vi "processScanCommand.vi"(8 "error in (no error)":errorcluster, 10 "Queues":T5, 11 "FPGA VI Reference In":T4) -> (0 "error out":errorcluster, 1 "command queue status":T1, 3 "num calls":T3, 4 "num lines sent":u32, 5 "num new volumes":i32, 6 "current volume":T2, 7 "line volume nums":i32[](array[numeric]))   [LabVIEW 2010]
uses:
  internal_queues.ctl
  line_info.ctl
  volume_with_lines.ctl
  volume_info.ctl
  FPGA_ref.ctl
  <vilib>/rvi/interface/nirviMethod/nirviMethod.xnode
  <vilib>/rvi/interface/common/niFpgaNodeNameForErrorReporting.ctl
  <vilib>/rvi/errors/niLvFpgaWhatHappensToTopLevelVI.ctl
  FPGA scanInfo/scan message.ctl
  <vilib>/Utility/error.llb/Error Cluster From Error Code.vi
  <vilib>/rvi/errors/niLvFpgaAdjustHostInterfaceError.vi
  NiFpgaLv.dll
panel:
  # "140 kHz * 2 = 280/ms"
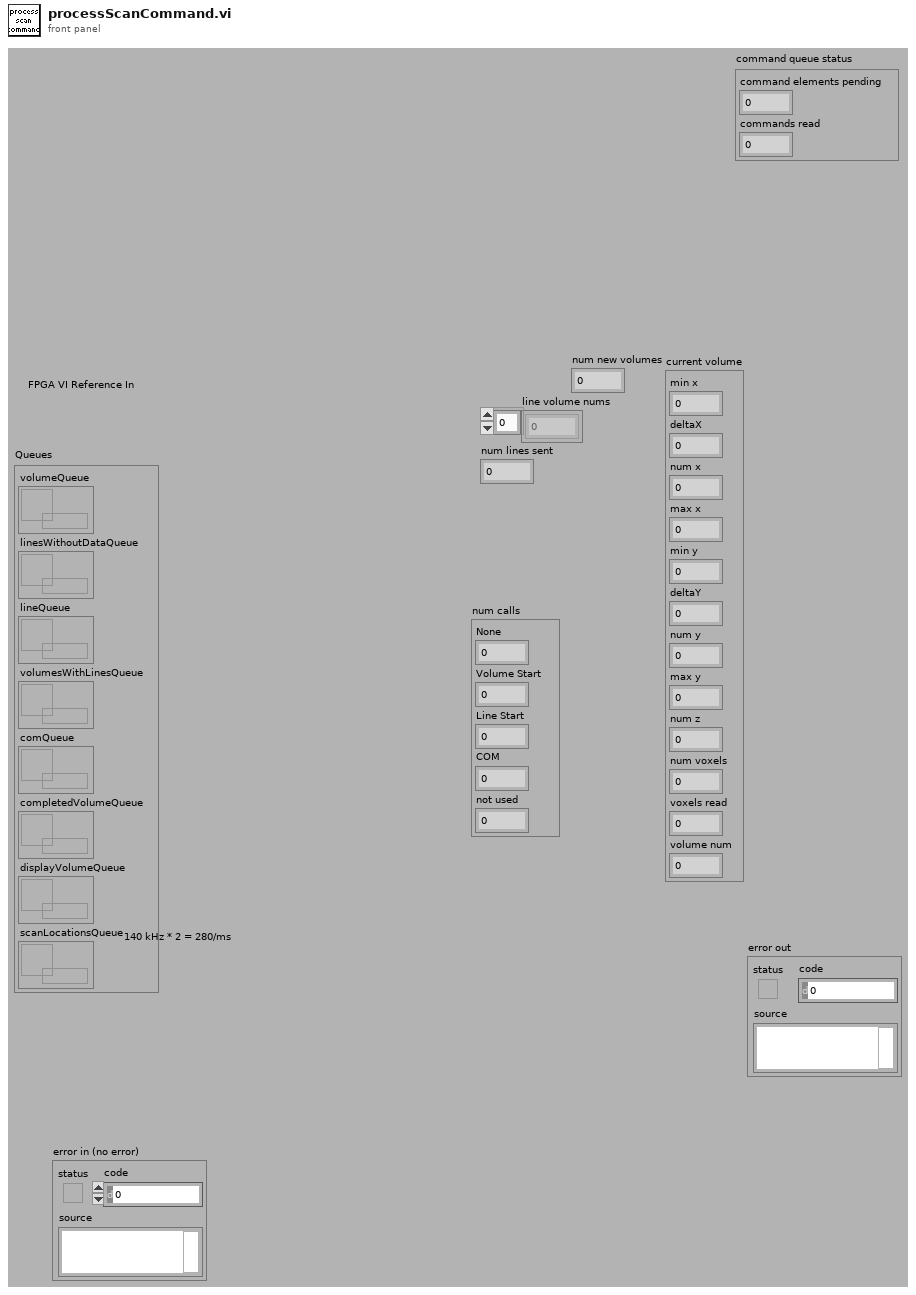
[diagram p1: front panel]
types:
  T1 = cluster{"command elements pending":u32, "commands read":u32}
  T2 = cluster{"min x":i16, "deltaX":dbl, "num x":u32, "max x":i16, "min y":i16, "deltaY":dbl, "num y":u32, "max y":i16, "num z":u32, "num voxels":u32, "voxels read":u32, "volume num":u32}
  T3 = cluster{"None":i32, "Volume Start":i32, "Line Start":i32, "COM":i32, "not used":i32}
  T4 = typedef "FPGA_ref.ctl" = refnum<k20>
  T5 = typedef "internal_queues.ctl" = cluster{"volumeQueue":refnum<queue>, "linesWithoutDataQueue":refnum<queue>, "lineQueue":refnum<queue>, "volumesWithLinesQueue":refnum<queue>, "comQueue":refnum<queue>, "completedVolumeQueue":refnum<queue>, "displayVolumeQueue":refnum<queue>, "scanLocationsQueue":refnum<queue>}
  T6 = cluster{"[0]":i32, "[1]":i32, "[2]":i32, "[3]":i32, "[4]":i32}
  T7 = typedef "scan message.ctl" = enum16{"NONE", "VOLUME START", "LINE START", "COM"}
  T8 = typedef "line_info.ctl" = cluster{"start X":i16, "start Y":i16, "start Z":i16, "end X":i16, "end Y":i16, "end Z":i16, "num z":u8, "voxel data":u32[], "volume num":u32, "line number":u16, "unused":u16}
  T9 = cluster{"Data[0]":i32, "Data[1]":i32, "Data[2]":i32, "Data[3]":i32, "Data[4]":i32}
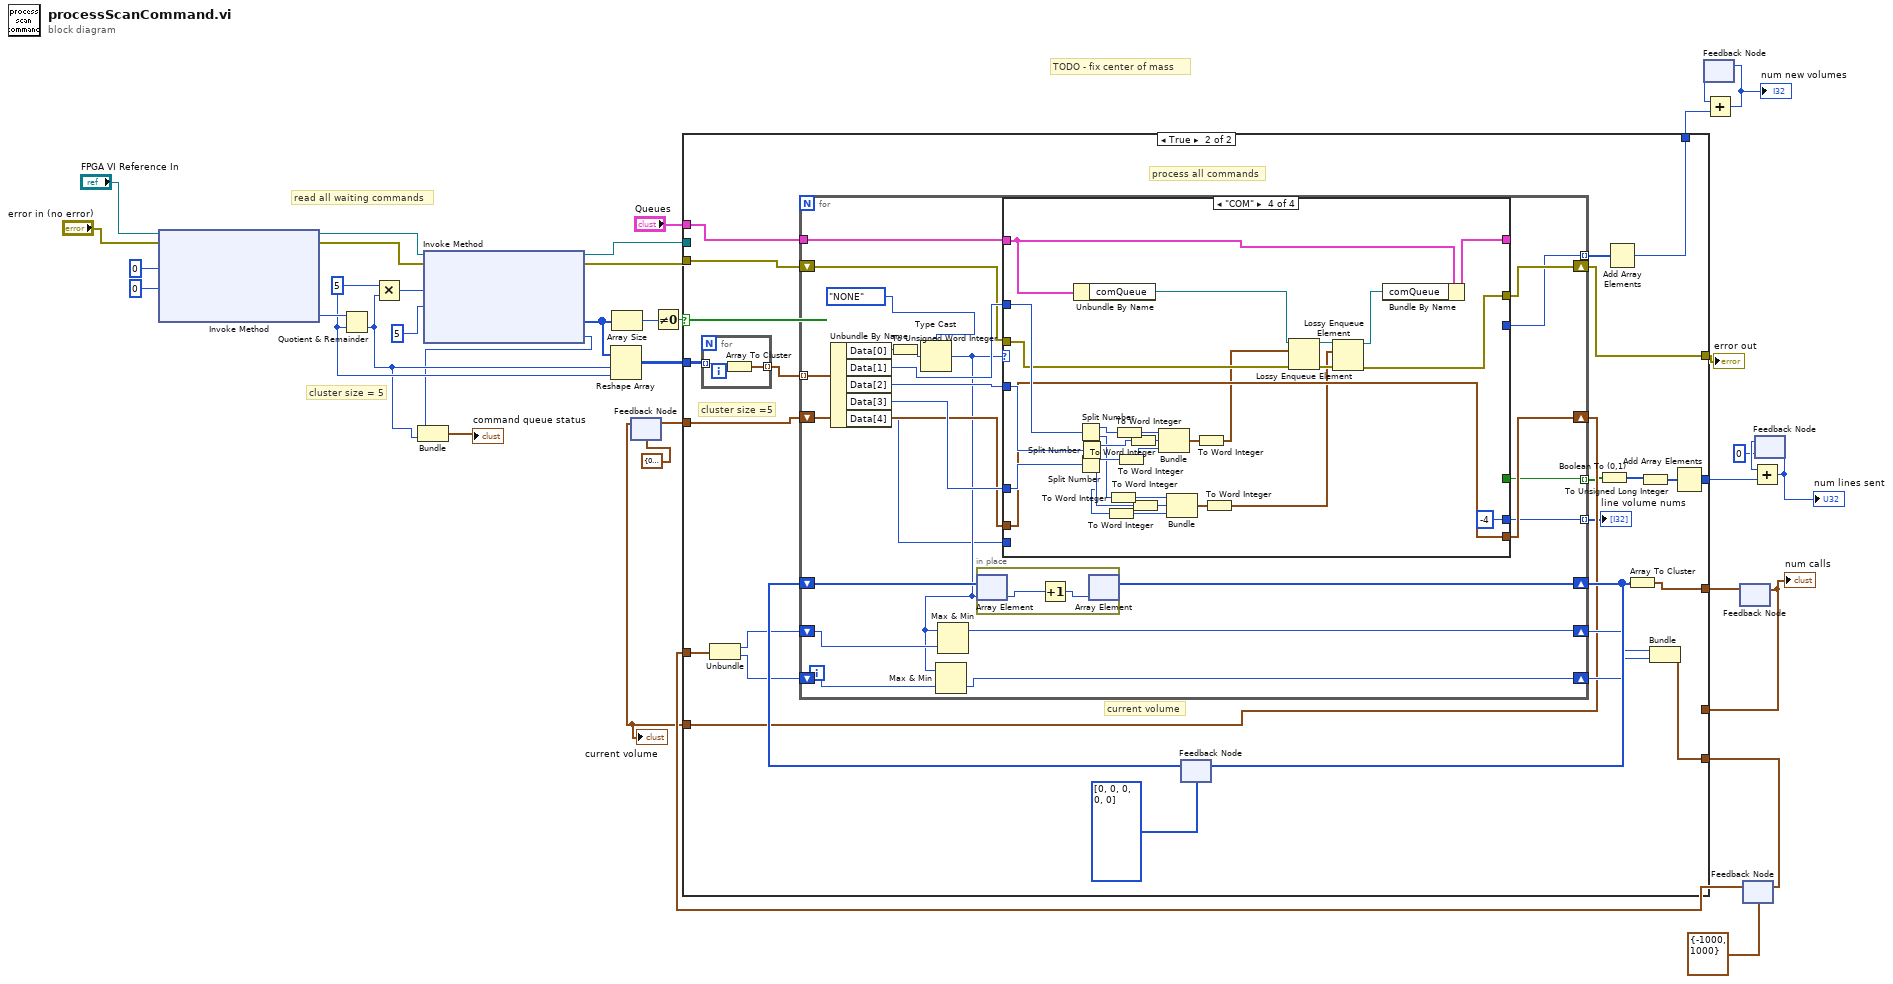
[diagram p0: block diagram]
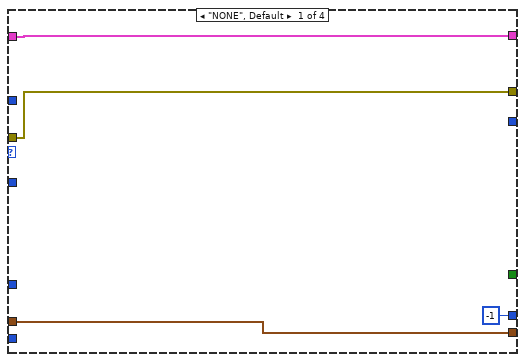
[diagram p3: hidden frame]
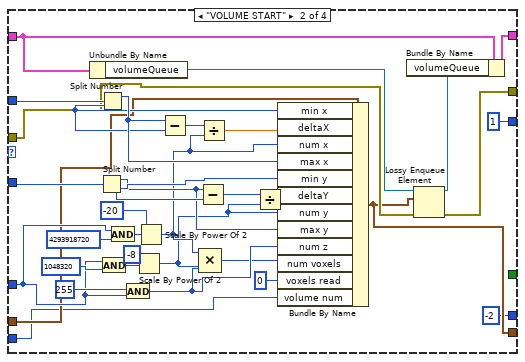
[diagram p4: hidden frame]
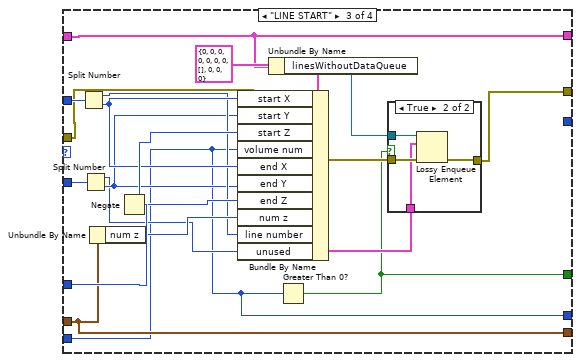
[diagram p5: hidden frame]
diagram:
  w24 = u32 5 ("Number of Elements")
  # "TODO - fix center of mass"
  # "read all waiting commands"
  # "cluster size = 5"
  n1 = xnode "Invoke Method"("FPGA VI Reference In"="FPGA VI Reference In", "error in"="error in (no error)", "Number of Elements"=u32 0, "Timeout (ms)"=0) -> ("FPGA VI Reference Out"=w22:T4, "error out"=w23:errorcluster, "Elements Remaining"=w25:u32)  [unwired: 1 out]
  n2 = Quotient & Remainder(x=w25, y=w24) -> (floor(x/y)=w6:u32)  [unwired: 1 out]
  n3 = Multiply(x=w24, y=w6) -> (x*y=w32:u32)
  n4 = xnode "Invoke Method"("FPGA VI Reference In"=w22, "error in"=w23, "Number of Elements"=w32, "Timeout (ms)"=5) -> ("FPGA VI Reference Out"=w33:T4, "error out"=w34:errorcluster, "Data"=w30:i32[], "Elements Remaining"=w5:u32)
  n5 = Bundle("Elements Remaining"=w5, w6) -> (→"command queue status":cluster{"Elements Remaining":u32, u32})  [unwired: 1 in]
  n6 = Reshape Array(w30, w6, w24) -> (w21:i32[][])
  n7 = Array Size(array=w30) -> (size(s)=w35:i32)
  n8 = feedback #1(T2 {"min x"=0, "deltaX"=0.0, "num x"=0, "max x"=0, "min y"=0, "deltaY"=0.0, "num y"=0, "max y"=0, "num z"=0, "num voxels"=0, "voxels read"=0, "volume num"=0} ("current volume")) -> (w9:T2)
  n9 = Not Equal To 0?(x=w35) -> (x != 0?=w31:bool)
  n10 = feedback #2() -> (w11:i32)  [unwired: 1 in]
  n11 = feedback #3() -> (w17:T6)  [unwired: 1 in]
  "num calls" <- w17
  n12 = feedback #4(cluster{i32, i32} {-1000, 1000}) -> (w16:cluster{i32, i32})
  n13 = case shown="True" w31 {
    tunnel: w34 -> [w40 w64]
    tunnel: w33 -> [_ _]
    tunnel: w21 -> [_ w63]
    tunnel: "Queues" -> [_ w61]
    tunnel: [w40 w46] -> w19
    tunnel: [w39 w57] -> w18
    tunnel: w17 -> [w39 _]
    tunnel: [w38 w54] -> w15
    tunnel: w16 -> [w38 w53]
    tunnel: [_ w49] -> w13
    tunnel: w9 -> [w37 w48]
    tunnel: [w37 w47] -> w8
    tunnel: [_ w41] -> w4
    frame False {
    }
    frame True {
      # "current volume"
      # "process all commands"
      # "cluster size =5"
      n14 = for {
        tunnel: w63 -> [w181] mode=indexing
        tunnel: [w180] -> w62 mode=indexing
        n15 = Array To Cluster(array=w181) -> (cluster=w180:T9)
      }
      n16 = Unbundle(w53) -> (w52:i32, w51:i32)
      n17 = feedback #5(i32[] [0, 0, 0, 0, 0]) -> (w60:i32[])
      n18 = for {
        tunnel: w62 -> [w67] mode=indexing
        shift-right: [w84] -> w46
        shift-left: w64 -> [w83]
        shift-right: [w81] -> w47
        shift-left: w48 -> [w80]
        shift-right: [w78] -> w58
        shift-left: w60 -> [w79]
        shift-right: [w76] -> w56
        shift-left: w52 -> [w75]
        shift-right: [w74] -> w55
        shift-left: w51 -> [w73]
        tunnel: [w72] -> w50 mode=indexing
        tunnel: w61 -> [w82]
        tunnel: [w66] -> w45 mode=indexing
        tunnel: [w65] -> w44 mode=indexing
        n19 = Unbundle By Name(w67) -> ("Data[0]"=w77:i32, "Data[1]"=w87:i32, "Data[2]"=w86:i32, "Data[3]"=w85:i32, "Data[4]"=w68:i32)
        n20 = To Unsigned Word Integer(number=w77) -> (unsigned 16bit integer=w70:u16)
        n21 = Type Cast(type=scan_message."NONE" ("Enum"), x=w70) -> (*(type *) &x=w71:T7)
        n22 = Max & Min(x=w71, y=w73) -> (min(x,y)=w74:i32)  [unwired: 1 out]
        n23 = Max & Min(x=w71, y=w75) -> (max(x,y)=w76:i32)  [unwired: 1 out]
        n24 = in-place {
          n25 = in-place-array #6(w79, w71) -> (w89:i32)
          n26 = Increment(x=w89) -> (x+1=w88:i32)
          n27 = in-place-array #6(w88) -> (w78:i32[])  [unwired: 1 out]
        }
        n28 = case shown="\"COM\"" w71 {
          tunnel: w87 -> [_ w127 w145 w178]
          tunnel: w86 -> [_ w126 w144 w177]
          tunnel: w85 -> [_ w122 w143 w176]
          tunnel: w82 -> [w93 w108 w138 w174]
          tunnel: w83 -> [w92 w110 w136 w171]
          tunnel: [w93 w106 w138 w173] -> _
          tunnel: [w92 w105 w135 w160] -> w84
          tunnel: [w91 w103 w141 w172] -> w81
          tunnel: w80 -> [w91 w104 w141 w172]
          tunnel: [_ 1 _ _] -> w72
          tunnel: w68 -> [_ w95 w129 _]
          tunnel: [-1 ("Data[4]") -2 ("Data[4]") w129 -4 ("Data[4]")] -> w66
          tunnel: [_ _ w128 _] -> w65
          frame "NONE", Default {
          }
          frame "VOLUME START" {
            n29 = Unbundle By Name(w108) -> ("volumeQueue"=w109:refnum<queue>)
            n30 = Split Number(x=w126) -> (hi(x)=w114:u16, lo(x)=w116:u16)
            n31 = Split Number(x=w127) -> (hi(x)=w119:u16, lo(x)=w118:u16)
            n32 = And(x=w122, y=u32 1048320) -> (x .and. y?=w98:u32)
            n33 = And(x=w122, y=u32 4293918720) -> (x .and. y?=w101:u32)
            n34 = And(x=u32 255, y=w122) -> (x .and. y?=w113:u32)
            n35 = Scale By Power Of 2(n=-8, x=w98) -> (x*2^n=w97:u32)
            n36 = Scale By Power Of 2(n=-20, x=w101) -> (x*2^n=w100:u32)
            n37 = Subtract(x=w119, y=w118) -> (x-y=w121:u16)
            n38 = Subtract(x=w114, y=w116) -> (x-y=w120:u16)
            n39 = Divide(x=w121, y=w100) -> (x/y=w117:dbl)
            n40 = Compound Arithmetic op=MULTIPLY(w100, w97, w113) -> (w112:u32)
            n41 = Divide(x=w120, y=w97) -> (x/y=w115:dbl)
            n42 = Bundle By Name(cluster=w104, "min x"=w118, "deltaX"=w117, "num x"=w100, "max x"=w119, "min y"=w116, "deltaY"=w115, "num y"=w97, "max y"=w114, "num z"=w113, "num voxels"=w112, "voxels read"=u32 0, "volume num"=w95) -> (w103:T2)
            n43 = Lossy Enqueue Element(queue=w109, element=w103, error in (no error)=w110) -> (queue out=w107:refnum<queue>, error out=w105:errorcluster)  [unwired: 2 out]
            n44 = Bundle By Name(cluster=w108, "volumeQueue"=w107) -> (w106:T5)
          }
          frame "LINE START" {
            n45 = Split Number(x=w145) -> (hi(x)=w132:u16, lo(x)=w133:u16)
            n46 = Split Number(x=w144) -> (hi(x)=w130:u16, lo(x)=w131:u16)
            n47 = Unbundle By Name(w141) -> ("num z"=w140:u32)
            n48 = Negate(x=w143) -> (-x=w142:i32)
            n49 = Bundle By Name(cluster=T8 {"start X"=0, "start Y"=0, "start Z"=0, "end X"=0, "end Y"=0, "end Z"=0, "num z"=0, "voxel data"=[], "volume num"=0, "line number"=0, "unused"=0} ("current line"), "start X"=w133, "start Y"=w131, "start Z"=w143, "volume num"=w129, "end X"=w133, "end Y"=w131, "end Z"=w142, "num z"=w140, "line number"=w132, "unused"=w130) -> (w134:T8)
            n50 = Unbundle By Name(w138) -> ("linesWithoutDataQueue"=w137:refnum<queue>)
            n51 = Greater Than 0?(x=w129) -> (x > 0?=w128:bool)
            n52 = case shown="True" w128 {
              tunnel: w137 -> [_ w150]
              tunnel: w136 -> [w146 w149]
              tunnel: [w146 w148] -> w135
              tunnel: w134 -> [_ w147]
              frame False {
              }
              frame True {
                n53 = Lossy Enqueue Element(queue=w150, element=w147, error in (no error)=w149) -> (error out=w148:errorcluster)  [unwired: 3 out]
              }
            }
          }
          frame "COM" {
            n54 = Unbundle By Name(w174) -> ("comQueue"=w175:refnum<queue>)
            n55 = Split Number(x=w178) -> (hi(x)=w169:u16, lo(x)=w164:u16)
            n56 = Split Number(x=w176) -> (hi(x)=w167:u16, lo(x)=w162:u16)
            n57 = Split Number(x=w177) -> (hi(x)=w168:u16, lo(x)=w163:u16)
            n58 = To Word Integer(number=w162) -> (16bit integer=w151:i16)
            n59 = To Word Integer(number=w164) -> (16bit integer=w153:i16)
            n60 = To Word Integer(number=w169) -> (16bit integer=w156:i16)
            n61 = To Word Integer(number=w167) -> (16bit integer=w154:i16)
            n62 = To Word Integer(number=w168) -> (16bit integer=w155:i16)
            n63 = To Word Integer(number=w163) -> (16bit integer=w152:i16)
            n64 = Bundle(w156, w155, w154) -> (w179:cluster{i16, i16, i16})  [unwired: 1 in]
            n65 = Bundle(w153, w152, w151) -> (w165:cluster{i16, i16, i16})  [unwired: 1 in]
            n66 = To Word Integer(number=w179) -> (16bit integer=w166:cluster{i16, i16, i16})
            n67 = To Word Integer(number=w165) -> (16bit integer=w157:cluster{i16, i16, i16})
            n68 = Lossy Enqueue Element(queue=w175, element=w166, error in (no error)=w171) -> (queue out=w158:refnum<queue>, error out=w161:errorcluster)  [unwired: 2 out]
            n69 = Lossy Enqueue Element(queue=w158, element=w157, error in (no error)=w161) -> (queue out=w159:refnum<queue>, error out=w160:errorcluster)  [unwired: 2 out]
            n70 = Bundle By Name(cluster=w174, "comQueue"=w159) -> (w173:T5)
          }
        }
      }
      "line volume nums" <- w45
      n71 = feedback-in #5(w58) -> ()
      n72 = Boolean To (0,1)(Boolean=w44) -> (0, 1=w43:i16[])
      n73 = Add Array Elements(numeric array=w50) -> (sum=w49:i32)
      n74 = Array To Cluster(array=w58) -> (cluster=w57:T6)
      n75 = To Unsigned Long Integer(number=w43) -> (unsigned 32bit integer=w42:u32[])
      n76 = Bundle(w56, w55) -> (w54:cluster{i32, i32})  [unwired: 1 in]
      n77 = Add Array Elements(numeric array=w42) -> (sum=w41:u32)
    }
  }
  "error out" <- w19
  "current volume" <- w8
  n78 = feedback-in #1(w8) -> ()
  n79 = Add(x=w11, y=w13) -> (x+y=w12:i32)
  "num new volumes" <- w12
  n80 = feedback-in #2(w12) -> ()
  n81 = feedback-in #3(w18) -> ()
  n82 = feedback-in #4(w15) -> ()
  n83 = feedback #7(u32 0) -> (w2:u32)
  n84 = Add(x=w2, y=w4) -> (x+y=w3:u32)
  "num lines sent" <- w3
  n85 = feedback-in #7(w3) -> ()
